vi "JTAG.vi"() -> ()   [LabVIEW 2021]
uses:
  controls/ID.ctl
panel:
  out "PWR error?":bool
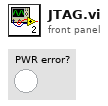
[diagram p1: front panel]
types:
  T1 = typedef "ID.ctl" = enum16{"1 - PWR", "2 - SM", "3 - DC", "4 - DM", "5 - WS", "6 - DS", "7 - WC", "8 - WA", "9 - WM", "10 - DA", "11 - WH", "12 - DH"}
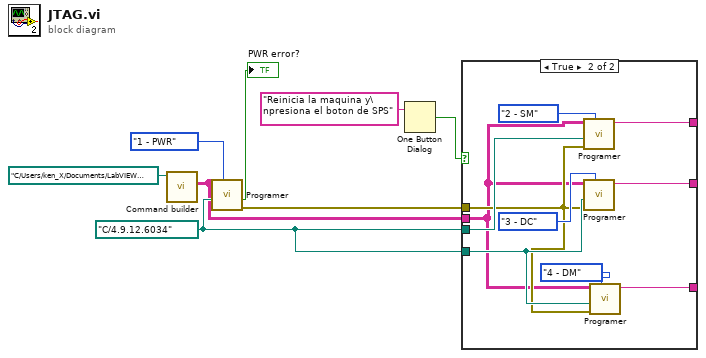
[diagram p0: block diagram]
diagram:
  w4 = path "C:/4.9.12.6034" ("configuration file path")
  n1 = call "Command builder.vi"("Config path"=path "C:/Users/ken_X/Documents/LabVIEW projects/Project-B2/settings/config.xls") -> ("Commands"=w3:string[][])  [unwired: 9 in, 1 out]
  n2 = call "Programer.vi"("ID"=ID."1 - PWR", "config path"=w4, "Commands"=w3) -> ("error out"=w5:errorcluster, "error?"=→"PWR error?":bool)  [unwired: 6 in, 1 out]
  n3 = One Button Dialog(message="Reinicia la maquina y\npresiona el boton de SPS") -> (true=w1:bool)  [unwired: 1 in]
  n4 = case shown="True" w1 {
    tunnel: w5 -> [_ w12]
    tunnel: w4 -> [_ w13]
    tunnel: w4 -> [_ w16]
    tunnel: w3 -> [_ w10]
    tunnel: [_ w15] -> _
    tunnel: [_ w14] -> _
    tunnel: [_ w11] -> _
    frame False {
    }
    frame True {
      n5 = call "Programer.vi"("ID"=ID."2 - SM", "error in"=w12, "config path"=w16, "Commands"=w10) -> ("Response"=w15:string)  [unwired: 5 in, 2 out]
      n6 = call "Programer.vi"("ID"=ID."3 - DC", "error in"=w12, "config path"=w13, "Commands"=w10) -> ("Response"=w14:string)  [unwired: 5 in, 2 out]
      n7 = call "Programer.vi"("ID"=ID."4 - DM", "error in"=w12, "config path"=w13, "Commands"=w10) -> ("Response"=w11:string)  [unwired: 5 in, 2 out]
    }
  }
